vi "testElementName.vi"(8 "error in (no error)":errorcluster, 11 "reference in":refnum<class "EasyXMLTest.lvclass">) -> (0 "error out":errorcluster, 3 "reference in":refnum<class "EasyXMLTest.lvclass">)   [LabVIEW 2013, in "EasyXMLTest.lvclass"]
uses:
  EasyXMLTest.lvclass
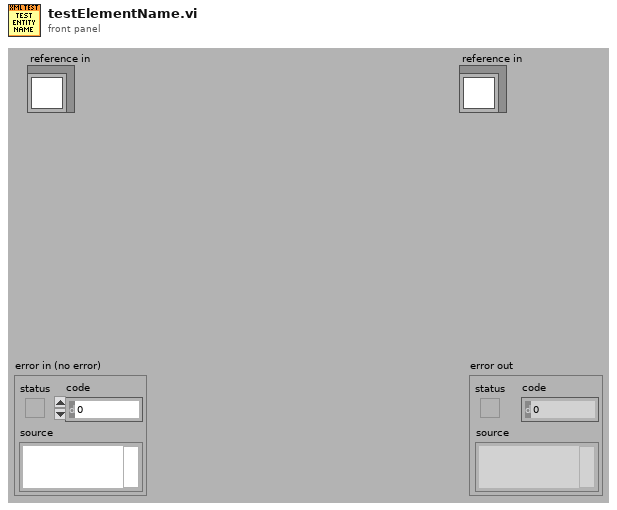
[diagram p1: front panel]
types:
  T1 = cluster{"LabVIEW data name":string, "xml element name":string}[]
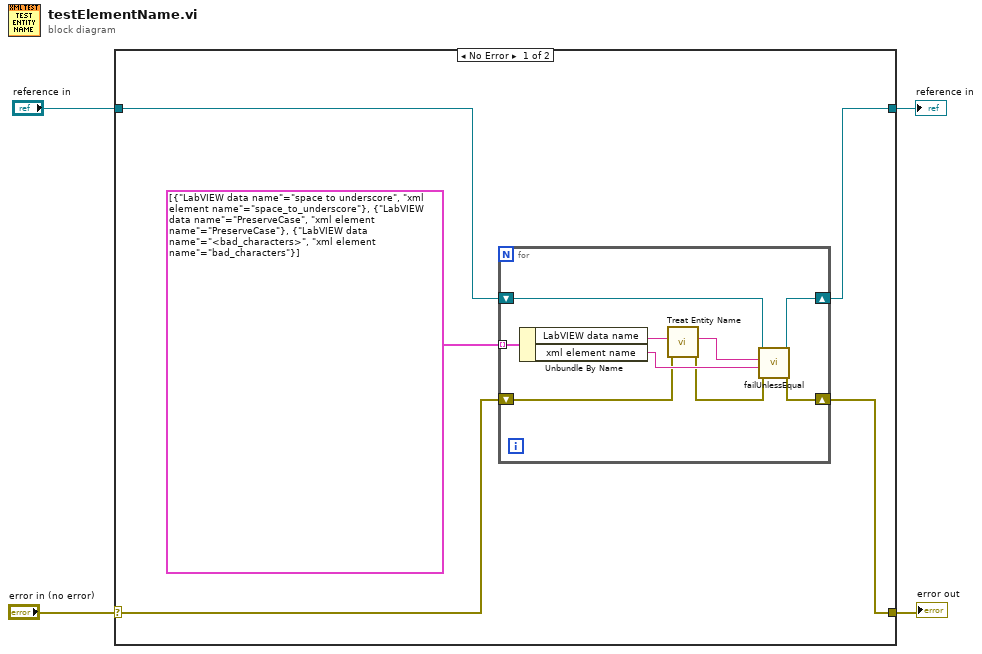
[diagram p0: block diagram]
diagram:
  n1 = case shown="No Error" "error in (no error)" {
    selector: "error in (no error)" -> [w8 w20]
    tunnel: [w7 w20] -> w3
    tunnel: [w5 w19] -> w1
    tunnel: "reference in" -> [w6 w19]
    frame No Error {
      n2 = for {
        tunnel: T1 [{"LabVIEW data name"="space to underscore", "xml element name"="space_to_underscore"}, {"LabVIEW data name"="PreserveCase", "xml element name"="PreserveCase"}, {"LabVIEW data name"="<bad_characters>", "xml element name"="bad_characters"}] -> [w18] mode=indexing
        shift-right: [w14] -> w7
        shift-left: w8 -> [w11]
        shift-right: [w13] -> w5
        shift-left: w6 -> [w12]
        n3 = Unbundle By Name(w18) -> ("LabVIEW data name"=w17:string, "xml element name"=w15:string)
        n4 = call "Treat Entity Name.vi"("error in"=w11, "Data Name"=w17) -> ("error out"=w10:errorcluster, "Entity Name"=w16:string)  [unwired: 7 in, 1 out]
        n5 = call-dynamic "failUnlessEqual.vi"("error in (no error)"=w10, "y"=w15, "x"=w16, "TestCase in"=w12) -> ("error out"=w14:errorcluster, "TestCase out"=w13:refnum<class "EasyXMLTest.lvclass">)  [unwired: 6 in]
      }
    }
    frame Error {
    }
  }
  "error out" <- w3
  "reference in" <- w1
